vi "Get State by Position.vi"(8 "error in (no error)":errorcluster, 10 "Position":u32, 11 "Example Application in":refnum<class "Example Application.lvclass">) -> (0 "error out":errorcluster, 2 "State":u32, 3 "Example Application out":refnum<class "Example Application.lvclass">)   [LabVIEW 2015, in "Example Application.lvlib" / "Example Application.lvclass"]
uses:
  Example Application.lvclass
  Example Application.lvclass/Example Application.ctl
  Properties/Example App Properties.lvclass
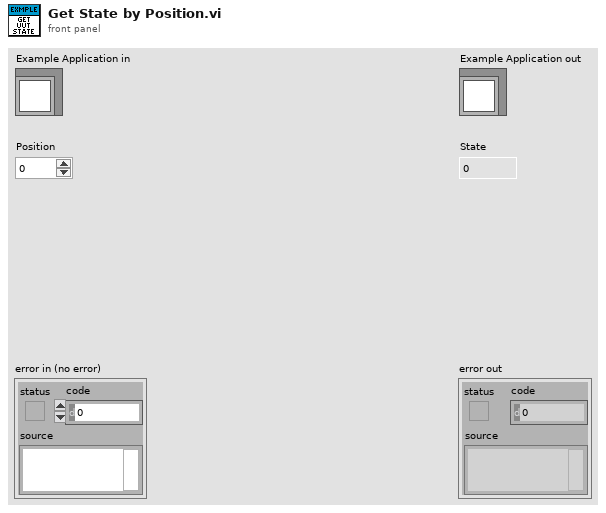
[diagram p1: front panel]
types:
  T1 = typedef "Example Application.lvlib/Example App Properties.lvclass/DUT State -- Enum.ctl" = enum16{"Idle", "Ready", "Testing", "Passed", "Failed"}
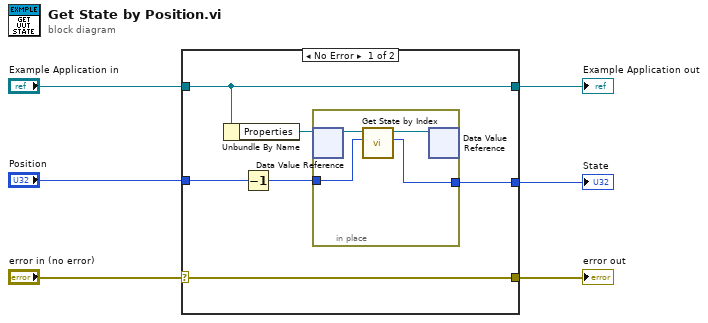
[diagram p0: block diagram]
diagram:
  n1 = case shown="No Error" "error in (no error)" {
    selector: "error in (no error)" -> [w9 w18]
    tunnel: "Example Application in" -> [w8 w17]
    tunnel: "Position" -> [w11 _]
    tunnel: [w9 w18] -> w4
    tunnel: [w8 w17] -> w1
    tunnel: [w7 _] -> w2
    frame No Error {
      n2 = Unbundle By Name(w8) -> ("Properties"=w12:refnum<data-value>)
      n3 = Decrement(x=w11) -> (x-1=w10:u32)
      n4 = in-place {
        in-place-border: w10 -> [w16]
        in-place-border: [w13] -> w7
        n5 = in-place-dvr #1(w12) -> (w15:refnum<class "Example App Properties.lvclass">)  [unwired: 1 out]
        n6 = call-dynamic "Get State by Index.vi"("index"=w16, "Example App Properties in"=w15) -> ("Enum"=w13:T1, "Example App Properties out"=w14:refnum<class "Example App Properties.lvclass">)  [unwired: 7 in, 1 out]
        n7 = in-place-dvr #1(w14) -> ()  [unwired: 2 out]
      }
    }
    frame Error {
    }
  }
  "error out" <- w4
  "Example Application out" <- w1
  "State" <- w2
